vi "Main.vi"(7 "mode":T1) -> ()   [LabVIEW 2020, in "InstrumentStudioPlugin_RenameMe.lvlib"]
doc: "This template is for the Queued Message Handler design pattern.\n\nThe Event Handling Loop generates messages based on user interface actions.\n\nThe Message Handling Loop processes messages generated by the Event Handling Loop, or by other messages. The messages are string values, so new messages can be added easily to the Message Cases case structure in the Message Handling Loop. Each message cluster can also provide an optional value for Message Data, which is a variant that can be converted to whatever message-specific data is required."
uses:
  InstrumentStudioPlugin_RenameMe.lvlib
  controls/Plugin Mode.ctl
  C:/Program Files/National Instruments/LabVIEW 2020/ProjectTemplates/Source/InstrumentStudioPlugin/PluginTemplate/subVIs/InstrumentStudioPlugin/InstrumentStudioPluginSDK.lvlibp/Plugin Events Enum.ctl
  controls/Configuration.ctl
  controls/Data.ctl
  Measurement Client Wrapper/Measurement Client Wrapper.lvclass
  controls/UI References.ctl
  Measurement Client Wrapper/Measurement Client Wrapper.lvclass/Measurement Client Wrapper.ctl
  Measurement Client Wrapper/Property/Read Display Name.vi
  Measurement Client Wrapper/Property/Read Version.vi
  subVIs/Message Queue/Enqueue Message (Single).vi
  subVIs/Message Queue/Enqueue Message (Array).vi
  <vilib>/Utility/error.llb/Error Cluster From Error Code.vi
  C:/Program Files/National Instruments/LabVIEW 2020/ProjectTemplates/Source/InstrumentStudioPlugin/PluginTemplate/subVIs/InstrumentStudioPlugin/InstrumentStudioPluginSDK.lvlibp/Read Run Time Configuration.vi
  C:/Program Files/National Instruments/LabVIEW 2020/ProjectTemplates/Source/InstrumentStudioPlugin/PluginTemplate/subVIs/InstrumentStudioPlugin/InstrumentStudioPluginSDK.lvlibp/Read Edit Time Configuration.vi
  C:/Program Files/National Instruments/LabVIEW 2020/ProjectTemplates/Source/InstrumentStudioPlugin/PluginTemplate/subVIs/InstrumentStudioPlugin/InstrumentStudioPluginSDK.lvlibp/Write Run Time Configuration.vi
  C:/Program Files/National Instruments/LabVIEW 2020/ProjectTemplates/Source/InstrumentStudioPlugin/PluginTemplate/subVIs/InstrumentStudioPlugin/InstrumentStudioPluginSDK.lvlibp/Write Edit Time Configuration.vi
  <vilib>/ErrorRing/Error Ring.xnode
  subVIs/Message Queue/Message Queue.lvlib
  subVIs/User Event - Stop/User Event - Stop.lvlib
  C:/Program Files/National Instruments/LabVIEW 2020/ProjectTemplates/Source/InstrumentStudioPlugin/PluginTemplate/subVIs/InstrumentStudioPlugin/InstrumentStudioPluginSDK.lvlibp/Plugin Session.lvclass
  C:/Program Files/National Instruments/LabVIEW 2020/ProjectTemplates/Source/InstrumentStudioPlugin/PluginTemplate/subVIs/InstrumentStudioPlugin/InstrumentStudioPluginSDK.lvlibp
panel:
  in  "Run Measurement":bool
  out "Version":string
  out "Measurement Name":string
  in  "Measurement Picker":bool
  out "Status":string
  in  "Read Run Time Config":bool
  in  "Read Edit Time Config":bool
  in  "Session Id":u64
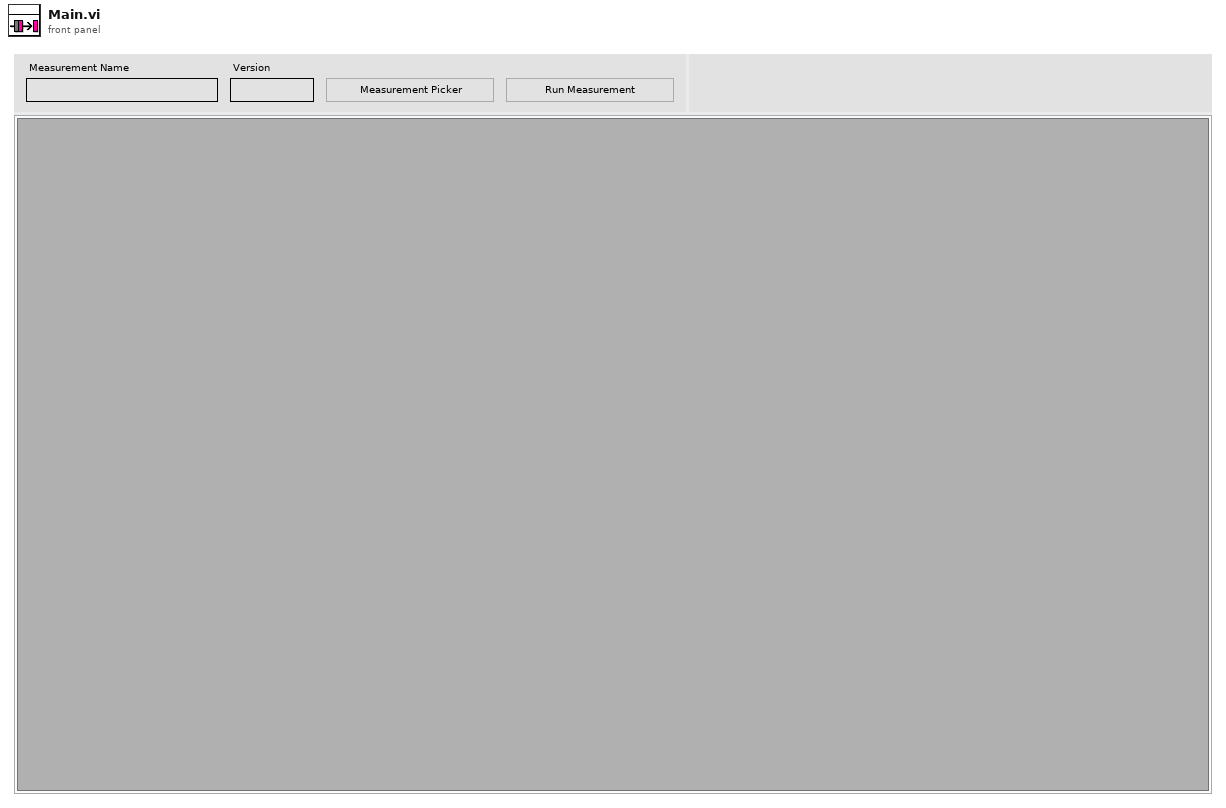
[diagram p1: front panel]
types:
  T1 = typedef "InstrumentStudioPlugin_RenameMe.lvlib/Plugin Mode.ctl" = enum16{"Interactive", "Automated"}
  T2 = typedef "InstrumentStudioPlugin_RenameMe.lvlib/UI References.ctl" = cluster{"UI Subpanel":refnum<vi>, "Status Message":string, "Matching UI & Meas Parameters?":bool}
  T3 = typedef "InstrumentStudioPlugin_RenameMe.lvlib/Data.ctl" = cluster{"Measurement Address":string, "Measurement Port":string, "Measurement Name":string, "Measurement Service":string, "Discovery Service address":string, "Measurement Service [obj]":refnum<class "Measurement Client Wrapper.lvclass">}
  T4 = typedef "InstrumentStudioPlugin_RenameMe.lvlib/Configuration.ctl" = cluster{"sample string":string}
  T5 = typedef "InstrumentStudioPluginSDK.lvlibp/Plugin Events Enum.ctl" = enum16{"Shutdown", "Project Saved", "Stop All Outputs"}
  T6 = typedef "InstrumentStudioPluginSDK.lvlibp/Event Registration Refnum.ctl" = refnum<event-registration>
  T7 = typedef "Message Queue.lvlib/All Message Queues.ctl" = cluster{"UI":refnum<queue>}
  T8 = cluster{"Event Refnum":T6, "Event Registration Refnum":refnum<event-registration>}
  T9 = enum8{"Enabled", "Disabled", "Disabled and Grayed Out"}
  T10 = cluster{"Measurement Name":string, "Measurement Service":string}
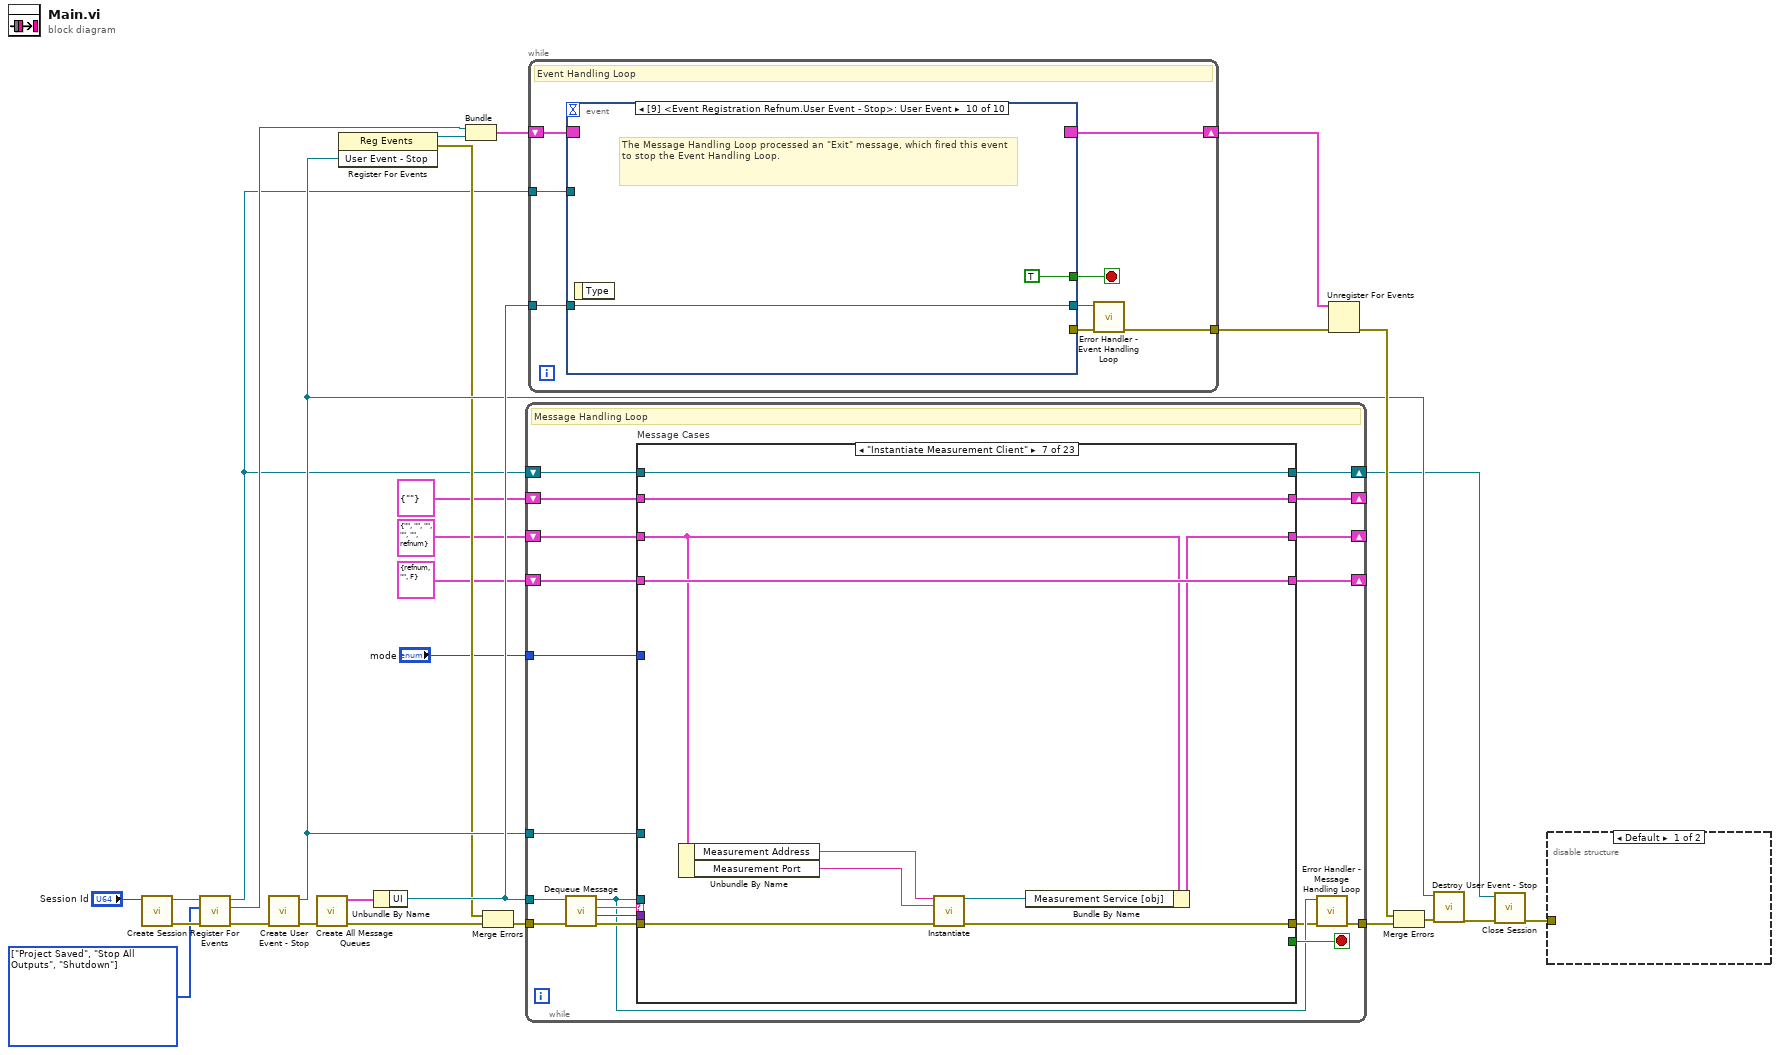
[diagram p0: block diagram]
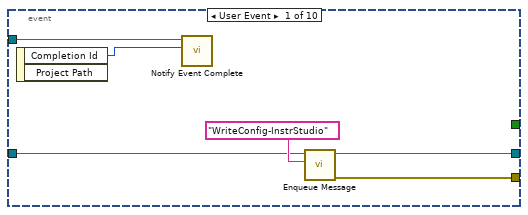
[diagram p3: hidden frame]
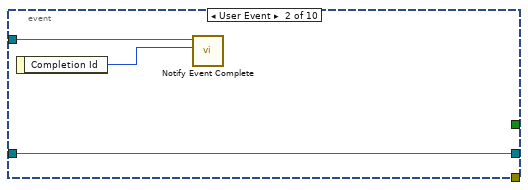
[diagram p4: hidden frame]
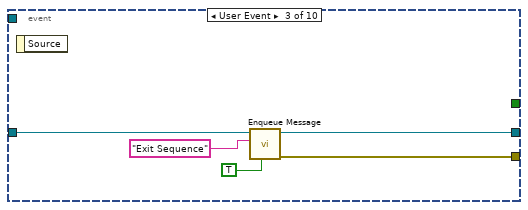
[diagram p5: hidden frame]
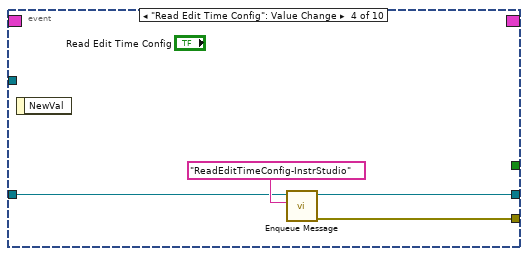
[diagram p6: hidden frame]
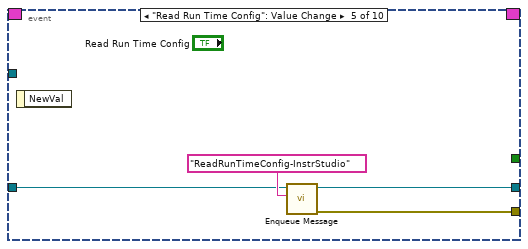
[diagram p7: hidden frame]
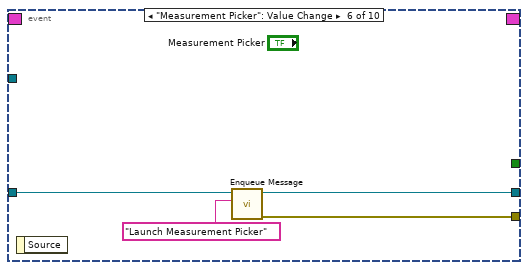
[diagram p8: hidden frame]
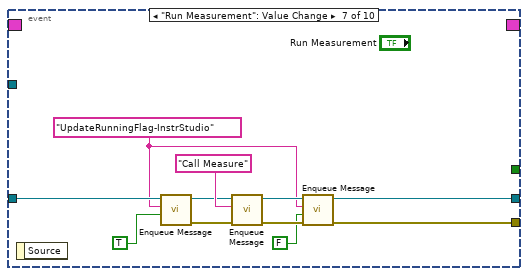
[diagram p9: hidden frame]
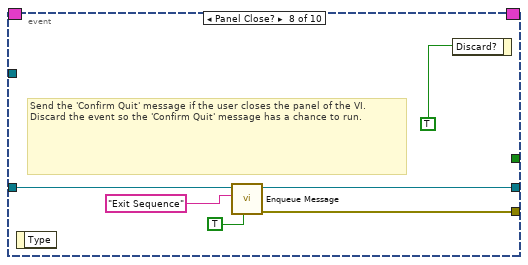
[diagram p10: hidden frame]
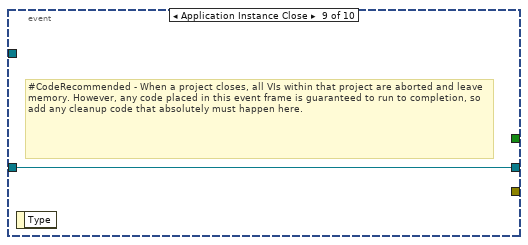
[diagram p11: hidden frame]
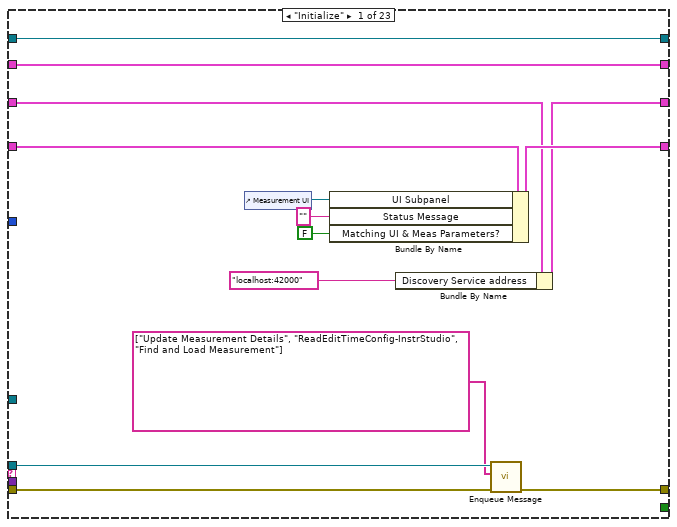
[diagram p12: hidden frame]
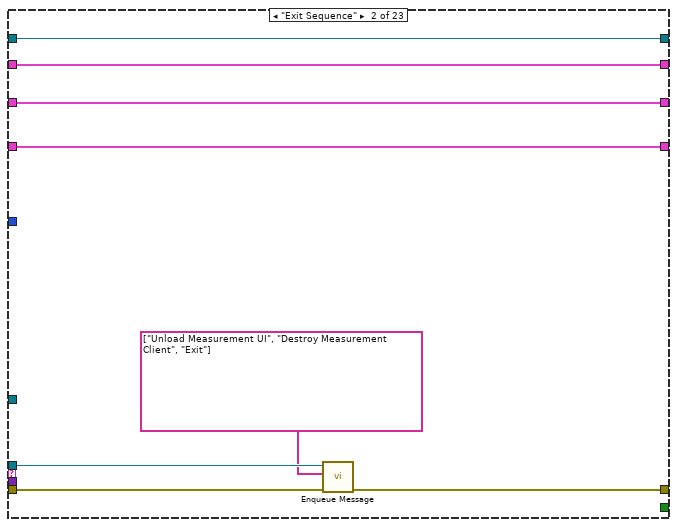
[diagram p13: hidden frame]
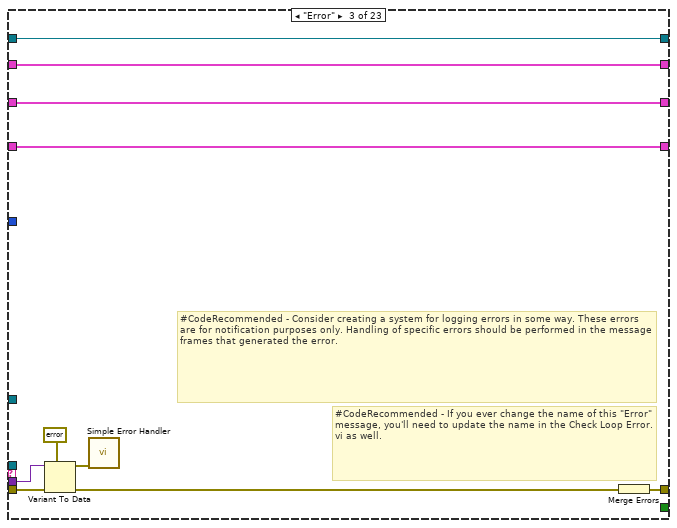
[diagram p14: hidden frame]
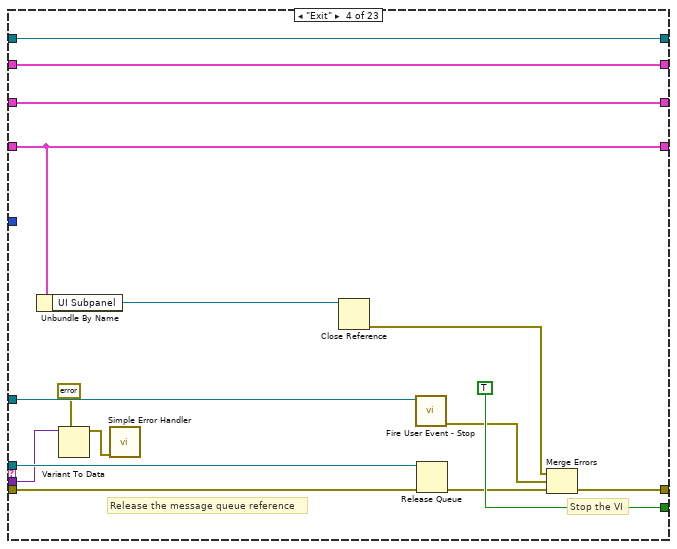
[diagram p15: hidden frame]
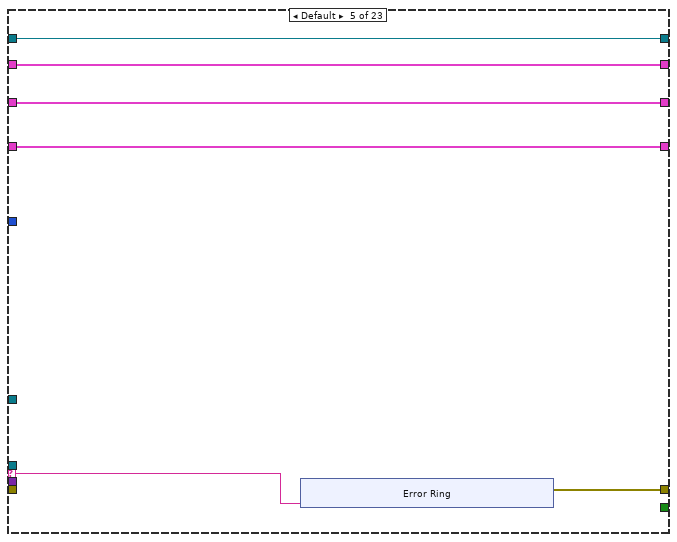
[diagram p16: hidden frame]
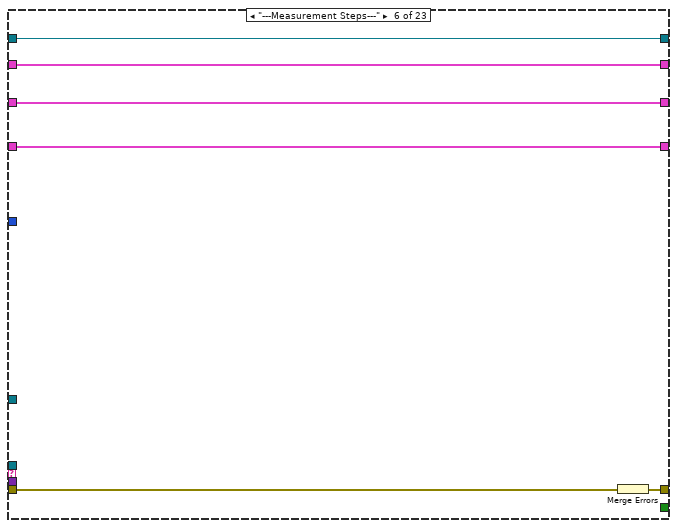
[diagram p17: hidden frame]
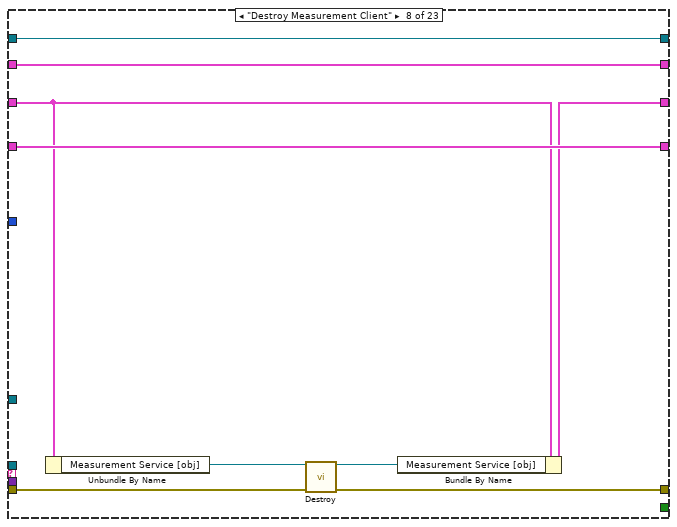
[diagram p18: hidden frame]
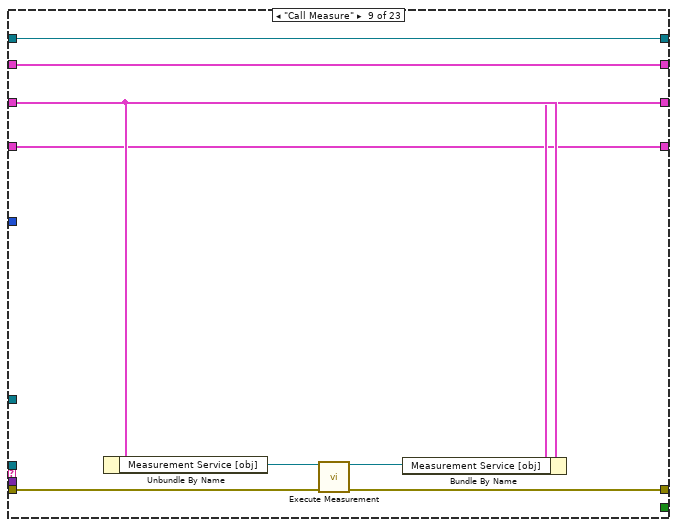
[diagram p19: hidden frame]
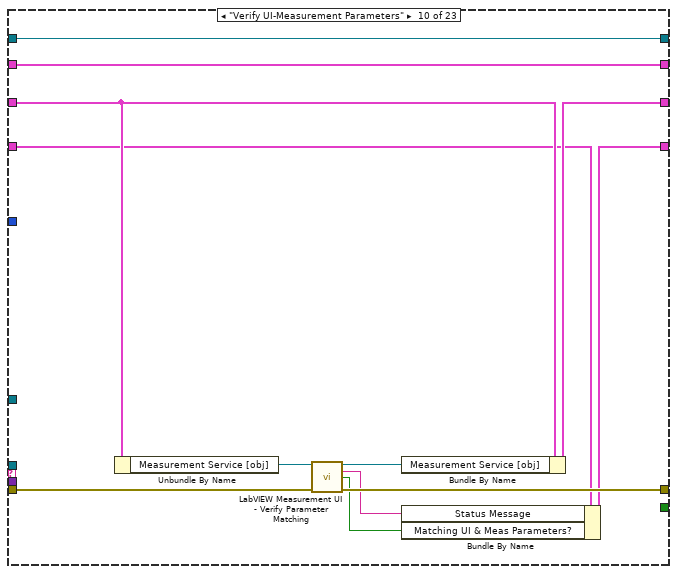
[diagram p20: hidden frame]
diagram:
  w12 = T5[] [enum."Project Saved", enum."Stop All Outputs", enum."Shutdown"] items=["Shutdown", "Project Saved", "Stop All Outputs"] ("Events To Register")
  n1 = call "Create Session.vi"("Session Id"="Session Id") -> ("error out"=w15:errorcluster, "Session out"=w13:refnum<class "Plugin Session.lvclass">)  [unwired: 6 in, 3 out]
  n2 = call "Register For Events.vi"("error in (no error)"=w15, "Events To Register"=w12, "Session in"=w13) -> ("error out"=w14:errorcluster, "Event Refnum"=w9:T6, "Session out"=w6:refnum<class "Plugin Session.lvclass">)  [unwired: 6 in]
  n3 = call "Create User Event - Stop.vi"("error in (no error)"=w14) -> ("error out"=w24:errorcluster, "User Event - Stop"=w19:refnum<user-event>)  [unwired: 9 in]
  n4 = call "Create All Message Queues.vi"("error in (no error)"=w24) -> ("error out"=w28:errorcluster, "Message Queues out"=w27:T7)  [unwired: 9 in]
  n5 = register-events(w19) -> (reference out=w11:refnum<event-registration>, error out=w17:errorcluster)  [unwired: 2 in]
  n6 = Unbundle By Name(w27) -> ("UI"=w25:refnum<queue>)
  n7 = Bundle("Event Refnum"=w9, "Event Registration Refnum"=w11) -> (w10:T8)  [unwired: 1 in]
  n8 = Merge Errors(w17, w28) -> (w18:errorcluster)
  n9 = while {
    tunnel: w25 -> [w39]
    shift-right: [w46] -> _
    shift-left: T3 {"Measurement Address"="", "Measurement Port"="", "Measurement Name"="", "Measurement Service"="", "Discovery Service address"="", "Measurement Service [obj]"=refnum} ("data") -> [w47]
    tunnel: w19 -> [w44]
    tunnel: w18 -> [w43]
    tunnel: [w37] -> w26
    shift-right: [w34] -> w8
    shift-left: w6 -> [w35]
    shift-right: [w33] -> _
    shift-left: T4 {"sample string"=""} ("Configuration") -> [w32]
    tunnel: "mode" -> [w31]
    shift-right: [w29] -> _
    shift-left: T2 {"UI Subpanel"=refnum, "Status Message"="", "Matching UI & Meas Parameters?"=FALSE} ("UI References") -> [w30]
    stop <- w45 stop-if-true
    # "Message Handling Loop"
    n10 = call "Dequeue Message.vi"("error in (no error)"=w43, "Message Queue"=w39) -> ("error out"=w42:errorcluster, "Message Data"=w40:variant, "Message"=w41:string, "dup Message Queue"=w38:refnum<queue>)  [unwired: 6 in]
    n11 = case "Message Cases" shown="\"Instantiate Measurement Client\"" w41 {
      selector: w41 -> [_ _ _ _ w99 _ _ _ _ _ _ _ _ _ _ _ _ _ _ _ _ _ _]
      tunnel: w38 -> [w52 w63 _ w95 _ _ _ _ _ _ _ w169 w196 _ _ _ _ _ _ _ _ _ _]
      tunnel: w42 -> [w54 w65 w79 w88 _ w114 w121 w130 w139 w147 w159 w171 w198 w216 w231 w242 w248 w263 w270 w279 w286 w301 w306]
      tunnel: [w53 w64 w73 w91 w100 w112 w120 w125 w136 w152 w159 w167 w194 w216 w219 w241 w247 w261 w271 w277 w285 w290 w315] -> w36
      tunnel: w47 -> [w56 w69 w78 w94 w101 w113 w115 w127 w138 w150 w158 w163 w190 w215 w232 w240 w251 w262 w274 w281 w284 w295 w311]
      tunnel: [w55 w69 w78 w94 w101 w113 w116 w128 w135 w151 w158 w164 w191 w215 w232 w239 w255 w262 w274 w281 w284 w291 w311] -> w46
      tunnel: [_ _ _ TRUE _ _ _ _ _ _ _ _ _ _ _ _ _ _ _ _ _ _ _] -> w45
      tunnel: w40 -> [_ _ w77 w85 _ _ _ _ _ _ _ _ _ _ _ _ _ _ w269 _ _ _ _]
      tunnel: w44 -> [_ _ _ w90 _ _ _ _ _ _ _ _ _ _ _ _ _ _ _ _ _ _ _]
      tunnel: w35 -> [w61 w68 w72 w84 w98 w111 w124 w133 w142 w154 w157 w174 w201 w214 w234 w244 w257 w260 w273 w280 w288 w303 w317]
      tunnel: [w61 w68 w72 w84 w98 w111 w124 w133 w142 w154 w157 w174 w201 w214 w234 w244 w257 w260 w272 w278 w287 w302 w316] -> w34
      tunnel: [w60 w67 w71 w83 w97 w110 w123 w132 w141 w153 w156 w173 w200 w213 w233 w243 w256 w259 w265 w276 w283 w300 w313] -> w33
      tunnel: w32 -> [w60 w67 w71 w83 w97 w110 w123 w132 w141 w153 w156 w173 w200 w213 w233 w243 w256 w259 w265 w276 w283 w300 w313]
      tunnel: w31 -> [_ _ _ _ _ _ _ _ _ _ _ _ _ _ _ _ _ _ _ _ _ _ _]
      tunnel: w30 -> [w59 w66 w70 w82 w96 w109 w122 w131 w134 w149 w155 w172 w199 w212 w224 w238 w254 w258 w264 w275 w282 w299 w312]
      tunnel: [w57 w66 w70 w82 w96 w109 w122 w131 w134 w148 w155 w172 w199 w212 w224 w238 w252 w258 w264 w275 w282 w299 w312] -> w29
      frame "Initialize" {
        # "Initialize - All initialization work should take place in this message, since other loops can potentially enqueue messages that execute immediately after this one."
        n12 = control-ref of="Measurement UI"() -> (w58:refnum<vi>)
        n13 = Bundle By Name(cluster=w59, "UI Subpanel"=w58, "Status Message"="", "Matching UI & Meas Parameters?"=FALSE) -> (w57:T2)
        n14 = Bundle By Name(cluster=w56, "Discovery Service address"="localhost:42000") -> (w55:T3)
        n15 = call-poly "Enqueue Message.vi"("error in (no error)"=w54, "Message Array"=string[] ["Update Measurement Details", "ReadEditTimeConfig-InstrStudio", "Find and Load Measurement"], "Message Queue"=w52) -> ("error out"=w53:errorcluster)  [unwired: 7 in, 1 out]
      }
      frame "Exit Sequence" {
        n16 = call-poly "Enqueue Message.vi"("error in (no error)"=w65, "Message Array"=string[] ["Unload Measurement UI", "Destroy Measurement Client", "Exit"], "Message Queue"=w63) -> ("error out"=w64:errorcluster)  [unwired: 7 in, 1 out]
      }
      frame "Error" {
        # "#CodeRecommended - If you ever change the name of this \"Error\" message, you'll need to update the name in the Check Loop Error.vi as well."
        # "#CodeRecommended - Consider creating a system for logging errors in some way. These errors are for notification purposes only. Handling of specific errors should be performed in the message frames that generated the error."
        # "Error - Display an error dialog. This message is sent by the \"Error Handler\" VIs at the end of other loops in this application."
        n17 = Variant To Data(error in=w79, type=errorcluster {"status"=FALSE, "code"=0, "source"=""} ("error constant"), Variant=w77) -> (data=w75:errorcluster, error out=w74:errorcluster)
        n18 = call <vilib>:"Simple Error Handler.vi"("error in (no error)"=w75) -> ()  [unwired: 4 in, 5 out]
        n19 = Merge Errors(w74) -> (w73:errorcluster)
      }
      frame "Exit" {
        # "Stop the VI"
        # "Release the message queue reference"
        # "Exit - Exit the application."
        n20 = Unbundle By Name(w82) -> ("UI Subpanel"=w81:refnum<vi>)
        n21 = Variant To Data(type=errorcluster {"status"=FALSE, "code"=0, "source"=""} ("error constant"), Variant=w85) -> (data=w86:errorcluster)  [unwired: 1 in, 1 out]
        n22 = call <vilib>:"Simple Error Handler.vi"("error in (no error)"=w86) -> ()  [unwired: 4 in, 5 out]
        n23 = Close Reference(reference=w81) -> (error out=w80:errorcluster)  [unwired: 1 in]
        n24 = call "Fire User Event - Stop.vi"("User Event - Stop"=w90) -> ("error out"=w89:errorcluster)  [unwired: 10 in]
        n25 = Release Queue(queue=w95, error in (no error)=w88) -> (error out=w92:errorcluster)  [unwired: 1 in, 2 out]
        n26 = Merge Errors(w80, w89, w92) -> (w91:errorcluster)
      }
      frame Default {
        # "'Default' case only runs if there is a message that isn't defined in any of the other cases.  Output a programming error."
        n27 = xnode "Error Ring"("parameter 0"=w99) -> ("error out"=w100:errorcluster)
      }
      frame "---Measurement Steps---" {
        # "Duplicate this frame when creating new messages.  Change this comment in the duplicated frame to describe this message."
        n28 = Merge Errors(w114) -> (w112:errorcluster)
      }
      frame "Instantiate Measurement Client" {
        n29 = Unbundle By Name(w115) -> ("Measurement Address"=w119:string, "Measurement Port"=w118:string)
        n30 = call "Instantiate.vi"("location"=w119, "insecurePort"=w118, "error in (no error)"=w121) -> ("Measurement Client Wrapper out"=w117:refnum<class "Measurement Client Wrapper.lvclass">, "error out"=w120:errorcluster)  [unwired: 11 in]
        n31 = Bundle By Name(cluster=w115, "Measurement Service [obj]"=w117) -> (w116:T3)
      }
      frame "Destroy Measurement Client" {
        n32 = Unbundle By Name(w127) -> ("Measurement Service [obj]"=w126:refnum<class "Measurement Client Wrapper.lvclass">)
        n33 = call "Destroy.vi"("Measurement Client Wrapper in"=w126, "error in"=w130) -> ("Measurement Client Wrapper out"=w129:refnum<class "Measurement Client Wrapper.lvclass">, "error out"=w125:errorcluster)  [unwired: 12 in]
        n34 = Bundle By Name(cluster=w127, "Measurement Service [obj]"=w129) -> (w128:T3)
      }
      frame "Call Measure" {
        n35 = Unbundle By Name(w138) -> ("Measurement Service [obj]"=w140:refnum<class "Measurement Client Wrapper.lvclass">)
        n36 = call "Execute Measurement.vi"("Measurement Client Wrapper"=w140, "error in"=w139) -> ("Measurement Client Wrapper out"=w137:refnum<class "Measurement Client Wrapper.lvclass">, "error out"=w136:errorcluster)  [unwired: 12 in]
        n37 = Bundle By Name(cluster=w138, "Measurement Service [obj]"=w137) -> (w135:T3)
      }
      frame "Verify UI-Measurement Parameters" {
        n38 = Unbundle By Name(w150) -> ("Measurement Service [obj]"=w146:refnum<class "Measurement Client Wrapper.lvclass">)
        n39 = call "LabVIEW Measurement UI - Verify Parameter Matching.vi"("Measurement Client Wrapper in"=w146, "error in"=w147) -> ("Measurement Client Wrapper"=w145:refnum<class "Measurement Client Wrapper.lvclass">, "Status"=w144:string, "Matching?"=w143:bool, "error out"=w152:errorcluster)  [unwired: 10 in]
        n40 = Bundle By Name(cluster=w150, "Measurement Service [obj]"=w145) -> (w151:T3)
        n41 = Bundle By Name(cluster=w149, "Status Message"=w144, "Matching UI & Meas Parameters?"=w143) -> (w148:T2)
      }
      frame "------Front Panel Interaction------" {
      }
      frame "Launch Measurement Picker" {
        n42 = Unbundle By Name(w163) -> ("Discovery Service address"=w162:string)
        n43 = call "Measurement Picker.vi"("discovery address"=w162, "error in"=w171) -> ("Cancelled?"=w170:bool, "Measurement location"=w166:string, "Measurement port"=w165:string, "Measurement Name"=w160:string, "Measurement Service"=w161:string, "error out"=w168:errorcluster)  [unwired: 8 in]
        n44 = case shown="False" w170 {
          tunnel: w169 -> [w184 _]
          tunnel: w168 -> [w183 w186]
          tunnel: [w182 w186] -> w167
          tunnel: w166 -> [w180 _]
          tunnel: w165 -> [w179 _]
          tunnel: w163 -> [w181 w185]
          tunnel: [w178 w185] -> w164
          tunnel: w161 -> [w176 _]
          tunnel: w160 -> [w175 _]
          frame False {
            n45 = Bundle By Name(cluster=w181, "Measurement Address"=w180, "Measurement Port"=w179, "Measurement Service"=w176, "Measurement Name"=w175) -> (w178:T3)
            n46 = call-poly "Enqueue Message.vi"("error in (no error)"=w183, "Message Array"=string[] ["Update Measurement Details", "Unload Measurement UI", "Destroy Measurement Client", "Instantiate Measurement Client", "Load Measurement UI", "Verify UI-Measurement Parameters", "Update Measurement Details", "WriteConfig-InstrStudio"], "Message Queue"=w184) -> ("error out"=w182:errorcluster)  [unwired: 7 in, 1 out]
          }
          frame True {
          }
        }
      }
      frame "Find and Load Measurement" {
        n47 = Unbundle By Name(w190) -> ("Discovery Service address"=w189:string, "Measurement Name"=w188:string, "Measurement Service"=w187:string)
        n48 = call "Discovery Service - Find Service.vi"("discovery address"=w189, "Measurement Name"=w188, "Measurement Service"=w187, "error in"=w198) -> ("Cancelled?"=w197:bool, "Measurement location"=w193:string, "Measurement port"=w192:string, "error out"=w195:errorcluster)  [unwired: 8 in]
        n49 = case shown="False" w197 {
          tunnel: w196 -> [w209 _]
          tunnel: w195 -> [w208 w211]
          tunnel: [w207 w211] -> w194
          tunnel: w193 -> [w205 _]
          tunnel: w192 -> [w204 _]
          tunnel: w190 -> [w206 w210]
          tunnel: [w203 w210] -> w191
          frame False {
            n50 = Bundle By Name(cluster=w206, "Measurement Address"=w205, "Measurement Port"=w204) -> (w203:T3)
            n51 = call-poly "Enqueue Message.vi"("error in (no error)"=w208, "Message Array"=string[] ["Unload Measurement UI", "Destroy Measurement Client", "Instantiate Measurement Client", "Load Measurement UI", "Verify UI-Measurement Parameters", "Update Measurement Details", "WriteConfig-InstrStudio"], "Message Queue"=w209) -> ("error out"=w207:errorcluster)  [unwired: 7 in, 1 out]
          }
          frame True {
          }
        }
      }
      frame "------Front Panel Updates------" {
      }
      frame "Update Measurement Details" {
        n52 = Unbundle By Name(w224) -> ("Status Message"=→"Status":string, "Matching UI & Meas Parameters?"=w217:bool)
        n53 = Unbundle By Name(w232) -> ("Measurement Service [obj]"=w222:refnum<class "Measurement Client Wrapper.lvclass">)
        n54 = Select(t=T9."Enabled" ("Disabled"), s=w217, f=T9."Disabled and Grayed Out" ("Disabled")) -> (s? t:f=w228:T9)
        n55 = property class="Measurement Client Wrapper.lvcl"(reference=w222) -> (error out=w218:errorcluster, "Property:Display Name"=→"Measurement Name":string, "Property:Version"=→"Version":string)  [unwired: 1 in, 1 out]
        n56 = property on="Run Measurement" class="Bool"(error in=w231, "DisabledEnum"=w228) -> (error out=w227:errorcluster)  [unwired: 1 in, 1 out]
        n57 = Not(x=w217) -> (.not. x?=w225:bool)
        n58 = property on="Status" class="Str"(error in=w227, "Visible"=w225) -> (error out=w226:errorcluster)  [unwired: 1 in, 1 out]
        n59 = Merge Errors(w226, w218) -> (w219:errorcluster)
      }
      frame "Load Measurement UI" {
        n60 = Unbundle By Name(w240) -> ("Measurement Service [obj]"=w236:refnum<class "Measurement Client Wrapper.lvclass">)
        n61 = Unbundle By Name(w238) -> ("UI Subpanel"=w235:refnum<vi>)
        n62 = call "LabVIEW Measurement UI - Open & Run.vi"("error in"=w242, "UI Subpanel"=w235, "Measurement Client Wrapper in"=w236) -> ("error out"=w241:errorcluster, "Measurement Client Wrapper"=w237:refnum<class "Measurement Client Wrapper.lvclass">)  [unwired: 6 in, 1 out]
        n63 = Bundle By Name(cluster=w240, "Measurement Service [obj]"=w237) -> (w239:T3)
      }
      frame "Unload Measurement UI" {
        n64 = Unbundle By Name(w251) -> ("Measurement Service [obj]"=w250:refnum<class "Measurement Client Wrapper.lvclass">)
        n65 = Unbundle By Name(w254) -> ("UI Subpanel"=w246:refnum<vi>)
        n66 = call "LabVIEW Measurement UI - Stop & Close.vi"("error in"=w248, "UI Subpanel"=w246, "Measurement Client Wrapper in"=w250) -> ("error out"=w247:errorcluster, "Measurement Client Wrapper"=w249:refnum<class "Measurement Client Wrapper.lvclass">)  [unwired: 7 in]
        n67 = Bundle By Name(cluster=w254, "Matching UI & Meas Parameters?"=FALSE, "Status Message"="") -> (w252:T2)
        n68 = Bundle By Name(cluster=w251, "Measurement Service [obj]"=w249) -> (w255:T3)
      }
      frame "---Instrument Studio Interaction---" {
        # "Duplicate this frame when creating new messages.  Change this comment in the duplicated frame to describe this message."
        n69 = Merge Errors(w263) -> (w261:errorcluster)
      }
      frame "UpdateRunningFlag-InstrStudio" {
        n70 = Variant To Data(error in=w270, type=TRUE, Variant=w269) -> (data=w267:bool, error out=w266:errorcluster)
        n71 = call "Update Running State.vi"("error in (no error)"=w266, "Is Running"=w267, "Plugin Session in"=w273) -> ("error out"=w271:errorcluster, "Plugin Session out"=w272:refnum<class "Plugin Session.lvclass">)  [unwired: 7 in]
      }
      frame "ReadISProjectPath" {
        n72 = call "Read Project Path.vi"("error in (no error)"=w279, "Session in"=w280) -> ("error out"=w277:errorcluster, "Session out"=w278:refnum<class "Plugin Session.lvclass">)  [unwired: 7 in, 1 out]
      }
      frame "ReadRunTimeConfig-InstrStudio" {
        n73 = property class="Plugin Session.lvclass" props=["Run Time Configuration"](reference=w288, error in=w286) -> (reference out=w287:refnum<class "Plugin Session.lvclass">, error out=w285:errorcluster)  [unwired: 1 out]
      }
      frame "ReadEditTimeConfig-InstrStudio" {
        w296 = T10 {"Measurement Name"="", "Measurement Service"=""}  # Config
        n74 = property class="Plugin Session.lvclass"(reference=w303, error in=w301) -> (reference out=w302:refnum<class "Plugin Session.lvclass">, error out=w297:errorcluster, "Edit Time Configuration"=w298:string)
        n75 = Unflatten From JSON(JSON string=w298, type and defaults=w296, error in (no error)=w297) -> (value=w294:T10, error out=w292:errorcluster)  [unwired: 4 in]
        n76 = Unbundle(w294) -> ("Measurement Name"=w293:string, "Measurement Service"=w289:string)
        n77 = call <vilib>:"Clear Errors.vi"("error in (no error)"=w292) -> ("error out"=w290:errorcluster)  [unwired: 5 in, 1 out]
        n78 = Bundle By Name(cluster=w295, "Measurement Name"=w293, "Measurement Service"=w289) -> (w291:T3)
      }
      frame "WriteConfig-InstrStudio" {
        w307 = T10 {"Measurement Name"="", "Measurement Service"=""}  # Config
        n79 = Unbundle By Name(w311) -> ("Measurement Name"=w310:string, "Measurement Service"=w309:string)
        n80 = Bundle(cluster=w307, "Measurement Name"=w310, "Measurement Service"=w309) -> (w308:T10)
        n81 = Flatten To JSON(anything=w308, error in (no error)=w306) -> (JSON string=w304:string, 11:w305:errorcluster)  [unwired: 1 in]
        n82 = property class="Plugin Session.lvclass"(reference=w317, error in=w305, "Run Time Configuration"="", "Edit Time Configuration"=w304) -> (reference out=w316:refnum<class "Plugin Session.lvclass">, error out=w315:errorcluster)
      }
    }
    n83 = call "Error Handler - Message Handling Loop.vi"("error in (no error)"=w36, "Message Queue"=w38) -> ("dup error in"=w37:errorcluster)  [unwired: 8 in, 1 out]
  }
  n84 = while {
    tunnel: w25 -> [w325]
    shift-right: [w323] -> w21
    shift-left: w10 -> [w324]
    tunnel: [w319] -> w20
    tunnel: w6 -> [w318]
    stop <- w321 stop-if-true
    # "Event Handling Loop"
    n85 = event shown="[9] <Event Registration Refnum.User Event - Stop>: User Event" {
      selector: w324 -> [_ _ _ _ _ _ _ _ _ _]
      dyn-events: [_ _ _ _ _ _ _ _ _ _] -> w323
      timeout: _ -> [_ _ _ _ _ _ _ _ _ _]
      tunnel: [_ _ _ _ _ _ _ _ _ TRUE ("Discard?")] -> w321
      tunnel: w325 -> [w328 w334 w337 w342 w346 w351 w361 w367 w369 w371]
      tunnel: [w326 _ w335 w340 w344 w348 w356 w366 _ _] -> w322
      tunnel: [w327 w334 w336 w341 w345 w350 w355 w365 w369 w371] -> w320
      tunnel: w318 -> [w331 w333 _ _ _ _ _ _ _ _]
      event User Event {
        n86 = event-data() -> ("Completion Id"=w330:i64)  [unwired: 1 in, 1 out]
        n87 = call "Notify Event Complete.vi"("Completion Id"=w330, "Session in"=w331) -> ()  [unwired: 8 in, 2 out]
        n88 = call-poly "Enqueue Message.vi"("Message"="WriteConfig-InstrStudio", "Message Queue"=w328) -> ("error out"=w326:errorcluster, "dup Message Queue"=w327:refnum<queue>)  [unwired: 8 in]
      }
      event User Event {
        n89 = event-data() -> ("Completion Id"=w332:i64)  [unwired: 1 in]
        n90 = call "Notify Event Complete.vi"("Completion Id"=w332, "Session in"=w333) -> ()  [unwired: 8 in, 2 out]
      }
      event User Event {
        n91 = event-data() -> ()  [unwired: 1 in, 1 out]
        n92 = call-poly "Enqueue Message.vi"("Priority Message? (F)"=TRUE, "Message"="Exit Sequence", "Message Queue"=w337) -> ("error out"=w335:errorcluster, "dup Message Queue"=w336:refnum<queue>)  [unwired: 7 in]
      }
      event "Read Edit Time Config": Value Change {
        n93 = event-data() -> ()  [unwired: 1 in, 1 out]
        n94 = call-poly "Enqueue Message.vi"("Message"="ReadEditTimeConfig-InstrStudio", "Message Queue"=w342) -> ("error out"=w340:errorcluster, "dup Message Queue"=w341:refnum<queue>)  [unwired: 8 in]
      }
      event "Read Run Time Config": Value Change {
        n95 = event-data() -> ()  [unwired: 1 in, 1 out]
        n96 = call-poly "Enqueue Message.vi"("Message"="ReadRunTimeConfig-InstrStudio", "Message Queue"=w346) -> ("error out"=w344:errorcluster, "dup Message Queue"=w345:refnum<queue>)  [unwired: 8 in]
      }
      event "Measurement Picker": Value Change {
        n97 = event-data() -> ()  [unwired: 1 in, 1 out]
        n98 = call-poly "Enqueue Message.vi"("Message"="Launch Measurement Picker", "Message Queue"=w351) -> ("error out"=w348:errorcluster, "dup Message Queue"=w350:refnum<queue>)  [unwired: 8 in]
      }
      event "Run Measurement": Value Change {
        w354 = "UpdateRunningFlag-InstrStudio" ("Message")
        n99 = event-data() -> ()  [unwired: 1 in, 1 out]
        n100 = call-poly "Enqueue Message.vi"("Message Data"=TRUE, "Message"=w354, "Message Queue"=w361) -> ("error out"=w359:errorcluster, "dup Message Queue"=w360:refnum<queue>)  [unwired: 7 in]
        n101 = call-poly "Enqueue Message.vi"("error in (no error)"=w359, "Message"="Call Measure", "Message Queue"=w360) -> ("error out"=w357:errorcluster, "dup Message Queue"=w358:refnum<queue>)  [unwired: 7 in]
        n102 = call-poly "Enqueue Message.vi"("error in (no error)"=w357, "Message Data"=FALSE, "Message"=w354, "Message Queue"=w358) -> ("error out"=w356:errorcluster, "dup Message Queue"=w355:refnum<queue>)  [unwired: 6 in]
      }
      event Panel Close? {
        # "Send the 'Confirm Quit' message if the user closes the panel of the VI. Discard the event so the 'Confirm Quit' message has a chance to run."
        n103 = event-data() -> ()  [unwired: 1 in, 1 out]
        n104 = call-poly "Enqueue Message.vi"("Priority Message? (F)"=TRUE, "Message"="Exit Sequence", "Message Queue"=w367) -> ("error out"=w366:errorcluster, "dup Message Queue"=w365:refnum<queue>)  [unwired: 7 in]
        n105 = event-data("Discard?"=TRUE) -> ()  [unwired: 1 in, 1 out]
      }
      event Application Instance Close {
        # "#CodeRecommended - When a project closes, all VIs within that project are aborted and leave memory. However, any code placed in this event frame is guaranteed to run to completion, so add any cleanup code that absolutely must happen here."
        n106 = event-data() -> ()  [unwired: 1 in, 1 out]
      }
      event User Event {
        # "The Message Handling Loop processed an \"Exit\" message, which fired this event to stop the Event Handling Loop."
        n107 = event-data() -> ()  [unwired: 1 in, 1 out]
      }
    }
    n108 = call "Error Handler - Event Handling Loop.vi"("error in (no error)"=w322, "Message Queue"=w320) -> ("dup error in"=w319:errorcluster)  [unwired: 8 in, 1 out]
  }
  n109 = Unregister For Events(event registration refnum=w21, error in=w20) -> (error out=w22:errorcluster)
  n110 = Merge Errors(w22, w26) -> (w23:errorcluster)
  n111 = call "Destroy User Event - Stop.vi"("error in (no error)"=w23, "User Event - Stop"=w19) -> ("error out"=w7:errorcluster)  [unwired: 9 in]
  n112 = call "Close Session.vi"("error in (no error)"=w7, "Session in"=w8) -> ("error out"=w1:errorcluster)  [unwired: 9 in]
  n113 = disable-structure shown="Default" {
    disable-tunnel: w1 -> [_ _]
    frame condition #0 (active) {
    }
    frame condition #1 {
      # "Call Quit LabVIEW if running as a built application."
    }
  }
